vi "SequenceRun.vi"(5 "EndTime":timestamp, 7 "StartTime":timestamp, 8 "error in":errorcluster, 11 "OperationRun":refnum<class "SequenceRun.lvclass">) -> (0 "error out":errorcluster, 3 "Passed":bool)   [LabVIEW 2020]
uses:
  ProligentResultProcessor/SequenceRun/SequenceRun/SequenceRun.lvclass
  ProligentResultProcessor/SequenceRun/SequenceRun/SetSequenceFullName.vi
  ProligentResultProcessor/SequenceRun/SequenceRun/SetStationFullName.vi
  ProligentResultProcessor/SequenceRun/SequenceRun/SetStartDate.vi
  ProligentResultProcessor/SequenceRun/SequenceRun/SetSequenceExecutionStatus.vi
  ProligentResultProcessor/SequenceRun/SequenceRun/SetEndDate.vi
  ProligentResultProcessor/SequenceRun/SequenceRun/SetSequenceRunId.vi
  ProligentResultProcessor/SequenceRun/SequenceRun/SetSequenceVersion.vi
  ProligentResultProcessor/SequenceRun/SequenceRun/SetUser.vi
  ProligentResultProcessor/SequenceRun/SequenceRun/GetSequenceFullName.vi
  ProligentResultProcessor/SequenceRun/SequenceRun/GetStationFullName.vi
  ProligentResultProcessor/SequenceRun/SequenceRun/GetStartDate.vi
  ProligentResultProcessor/SequenceRun/SequenceRun/GetSequenceExecutionStatus.vi
  ProligentResultProcessor/SequenceRun/SequenceRun/GetEndDate.vi
  ProligentResultProcessor/SequenceRun/SequenceRun/GetSequenceRunId.vi
  ProligentResultProcessor/SequenceRun/SequenceRun/GetSequenceVersion.vi
  ProligentResultProcessor/SequenceRun/SequenceRun/GetUser.vi
  ProligentResultProcessor/SequenceRun/SequenceRun/GetStepRuns.vi
  ProligentResultProcessor/SequenceRun/SequenceRun/GetCharacteristics.vi
  ProligentResultProcessor/SequenceRun/SequenceRun/GetDocuments.vi
  ProligentResultProcessor/SequenceRun/SequenceRun/GetFailureReferences.vi
  ProligentResultProcessor/SequenceRun/SequenceRun/GetCustomData.vi
  ProligentResultProcessor/StepRun/StepRun/StepRun.lvclass
  ProligentResultProcessor/Model/Characteristic/Characteristic.lvclass
  ProligentResultProcessor/Model/Document/Document.lvclass
  ProligentResultProcessor/Failure/FailureReference/FailureReference.lvclass
  ProligentResultProcessor/Model/CustomData/CustomData.lvclass
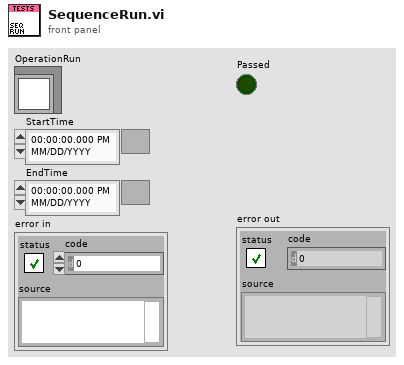
[diagram p1: front panel]
types:
  T1 = enum16{"PASS", "FAIL", "NOT_COMPLETED", "ABORTED"}
  T2 = typedef "ProligentResultProcessor.lvlib/ExecutionStatus.lvclass/Value.ctl" = enum16{"PASS", "FAIL", "NOT_COMPLETED", "ABORTED"}
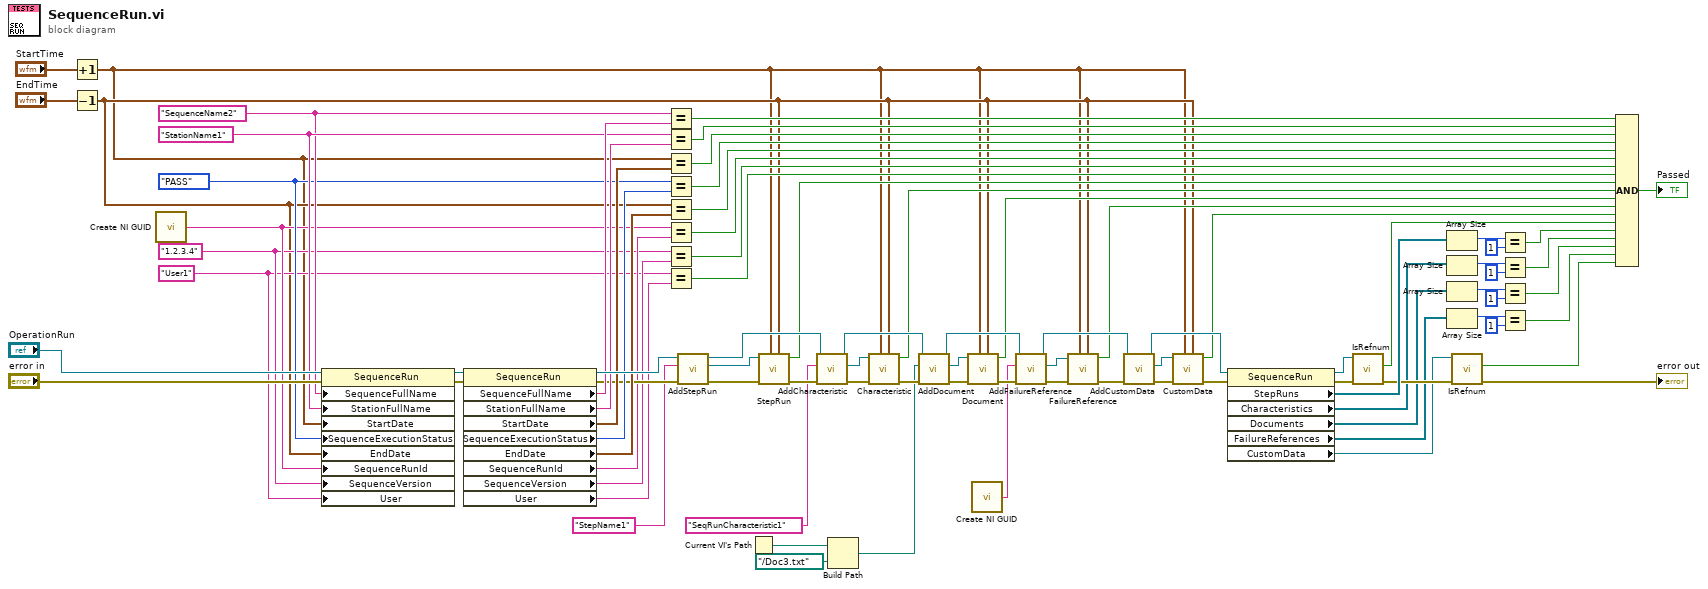
[diagram p0: block diagram]
diagram:
  w5 = "User1"
  w10 = "1.2.3.4"
  w64 = T1."PASS" ("ProcessRunStatus")
  w77 = "StationName1"
  w76 = "SequenceName2"
  n1 = Increment(x="StartTime") -> (x+1=w1:timestamp)
  n2 = Decrement(x="EndTime") -> (x-1=w2:timestamp)
  n3 = call <vilib>:"Create NI GUID.vi"() -> ("NI GUID"=w14:string)
  n4 = property class="SequenceRun"(reference="OperationRun", error in="error in", "SequenceFullName"=w76, "StationFullName"=w77, "StartDate"=w1, "SequenceExecutionStatus"=w64, "EndDate"=w2, "SequenceRunId"=w14, "SequenceVersion"=w10, "User"=w5) -> (reference out=w84:refnum<class "SequenceRun.lvclass">, error out=w83:errorcluster)
  n5 = property class="SequenceRun"(reference=w84, error in=w83) -> (reference out=w87:refnum<class "SequenceRun.lvclass">, error out=w75:errorcluster, "SequenceFullName"=w82:string, "StationFullName"=w81:string, "StartDate"=w80:timestamp, "SequenceExecutionStatus"=w79:T2, "EndDate"=w78:timestamp, "SequenceRunId"=w13:string, "SequenceVersion"=w9:string, "User"=w4:string)
  n6 = Equal?(x=w76, y=w82) -> (x = y?=w70:bool)
  n7 = Equal?(x=w77, y=w81) -> (x = y?=w69:bool)
  n8 = Equal?(x=w1, y=w80) -> (x = y?=w68:bool)
  n9 = Equal?(x=w64, y=w79) -> (x = y?=w67:bool)
  n10 = Equal?(x=w2, y=w78) -> (x = y?=w15:bool)
  n11 = Equal?(x=w14, y=w13) -> (x = y?=w12:bool)
  n12 = Equal?(x=w10, y=w9) -> (x = y?=w11:bool)
  n13 = Equal?(x=w5, y=w4) -> (x = y?=w3:bool)
  n14 = call "AddStepRun.vi"("error in"=w75, "StepName"="StepName1", "SequenceRun in"=w87) -> ("error out"=w59:errorcluster, "StepRun"=w58:refnum<class "StepRun.lvclass">, "SequenceRun out"=w60:refnum<class "SequenceRun.lvclass">)  [unwired: 6 in]
  n15 = Current VI's Path() -> (path=w8:path)
  n16 = call "StepRun.vi"("EndTime"=w2, "StartTime"=w1, "error in"=w59, "StepRun"=w58) -> ("error out"=w53:errorcluster, "Passed"=w41:bool)  [unwired: 6 in]
  n17 = call "AddCharacteristic.vi"("error in"=w53, "FullName"="SeqRunCharacteristic1", "SequenceRun in"=w60) -> ("error out"=w52:errorcluster, "Characteristic"=w51:refnum<class "Characteristic.lvclass">, "SequenceRun out"=w54:refnum<class "SequenceRun.lvclass">)  [unwired: 6 in]
  n18 = Build Path(base path=w8, name or relative path=path "../Doc3.txt" ("FilePath")) -> (appended path=w6:path)
  n19 = call "Characteristic.vi"("EndTime"=w2, "StartTime"=w1, "error in (no error)"=w52, "Characteristic in"=w51) -> ("error out"=w48:errorcluster, "Passed"=w40:bool)  [unwired: 6 in]
  n20 = call "AddDocument.vi"("error in"=w48, "FilePath"=w6, "SequenceRun in"=w54) -> ("error out"=w47:errorcluster, "Document"=w46:refnum<class "Document.lvclass">, "SequenceRun out"=w49:refnum<class "SequenceRun.lvclass">)  [unwired: 6 in]
  n21 = call "Document.vi"("EndTime"=w2, "StartTime"=w1, "error in (no error)"=w47, "Characteristic in"=w46) -> ("error out"=w44:errorcluster, "Passed"=w39:bool)  [unwired: 6 in]
  n22 = call <vilib>:"Create NI GUID.vi"() -> ("NI GUID"=w17:string)
  n23 = call "AddFailureReference.vi"("error in"=w44, "Id"=w17, "SequenceRun in"=w49) -> ("error out"=w43:errorcluster, "Document"=w42:refnum<class "FailureReference.lvclass">, "SequenceRun out"=w45:refnum<class "SequenceRun.lvclass">)  [unwired: 6 in]
  n24 = call "FailureReference.vi"("EndTime"=w2, "StartTime"=w1, "error in"=w43, "Defect"=w42) -> ("error out"=w36:errorcluster, "Passed"=w38:bool)  [unwired: 6 in]
  n25 = call "AddCustomData.vi"("error in"=w36, "SequenceRun in"=w45) -> ("error out"=w35:errorcluster, "CustomData"=w33:refnum<class "CustomData.lvclass">, "SequenceRun out"=w37:refnum<class "SequenceRun.lvclass">)  [unwired: 7 in]
  n26 = call "CustomData.vi"("EndTime"=w2, "StartTime"=w1, "error in"=w35, "CustomData"=w33) -> ("error out"=w34:errorcluster, "Passed"=w16:bool)  [unwired: 6 in]
  n27 = property class="SequenceRun"(reference=w37, error in=w34) -> (reference out=w56:refnum<class "SequenceRun.lvclass">, error out=w71:errorcluster, "StepRuns"=w72:refnum<class "StepRun.lvclass">[], "Characteristics"=w26:refnum<class "Characteristic.lvclass">[], "Documents"=w25:refnum<class "Document.lvclass">[], "FailureReferences"=w24:refnum<class "FailureReference.lvclass">[], "CustomData"=w19:refnum<class "CustomData.lvclass">)
  n28 = call "IsRefnum.vi"("error in"=w71, "SequenceRun in"=w56) -> ("error out"=w57:errorcluster, "IsRefnum"=w55:bool)  [unwired: 7 in, 1 out]
  n29 = Array Size(array=w72) -> (size(s)=w74:i32)
  n30 = Array Size(array=w26) -> (size(s)=w31:i32)
  n31 = Array Size(array=w25) -> (size(s)=w30:i32)
  n32 = Array Size(array=w24) -> (size(s)=w27:i32)
  n33 = call "IsRefnum.vi"("error in"=w57, "CustomDataType in"=w19) -> ("error out"=→"error out":errorcluster, "IsRefnum"=w18:bool)  [unwired: 7 in, 1 out]
  n34 = Equal?(x=w74, y=1) -> (x = y?=w66:bool)
  n35 = Equal?(x=w31, y=1) -> (x = y?=w23:bool)
  n36 = Equal?(x=w30, y=1) -> (x = y?=w22:bool)
  n37 = Equal?(x=w27, y=1) -> (x = y?=w21:bool)
  n38 = Compound Arithmetic op=AND(w70, w69, w68, w67, w15, w12, w11, w3, w41, w40, w39, w38, w16, w55, w66, w23, w22, w21, w18) -> (→"Passed":bool)
